vi "LINC Write Command.vi"(6 "timeout (2000)":u32=2000, 7 "parse only (F)":bool, 8 "error in (no error)":errorcluster, 9 "string command":string, 10 "packet":variant, 11 "LINC session":refnum<class "LINC.lvclass">) -> (0 "error out":errorcluster, 1 "remote error":bool, 2 "binary command":string, 3 "dup LINC session":refnum<class "LINC.lvclass">)   [LabVIEW 2018, in "STEPkgDriver_LINC.lvlib" / "LINC.lvclass"]
uses:
  LINC.lvclass
  STEPkgDriver_LINC.lvlib
  LINC Global Mode.ctl
  LINC Global Session Mode.ctl
  LINC Global Config Mode.ctl
  LINC Global Handshake Mode.ctl
  LINC Handshake Internal.ctl
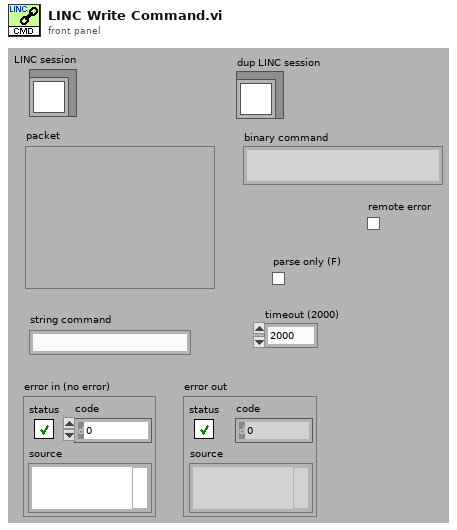
[diagram p1: front panel]
types:
  T1 = typedef "STEPkgDriver_LINC.lvlib/LINC Global Config Mode.ctl" = enum16{"INIT", "CLEAR", "SET_CMD_CB", "SET_TLM_CB", "SET_CMD_FIELDS", "SET_TLM_FIELDS", "SET_ID", "GET_CONFIG"}
  T2 = typedef "STEPkgDriver_LINC.lvlib/LINC Global Mode.ctl" = enum16{"INIT", "CLEAR", "ADD_PKT_HDR", "ADD_PKT", "GET_PKT_NAMES", "GET_PKT_DESC", "GET_PKT_HDR", "GET_PKT", "SET_PKT", "SET_DATA", "SIM_EN", "SIM_DS"}
  T3 = typedef "STEPkgDriver_LINC.lvlib/LINC Handshake Internal.ctl" = cluster{"error":errorcluster, "command data":string}
  T4 = typedef "STEPkgDriver_LINC.lvlib/LINC Global Handshake Mode.ctl" = enum16{"INIT", "CLEAR", "ADD_COMMAND", "RMV_COMMAND", "CLR_HANDSHAKE", "SET_HANDSHAKE", "GET_HANDSHAKE"}
  T5 = typedef "STEPkgDriver_LINC.lvlib/LINC Global Session Mode.ctl" = enum16{"INIT", "CLEAR", "ADD_SESSION", "SET_CONNECTION", "SET_LISTENER", "SET_REFERENCE", "GET_SESSION"}
  T6 = typedef "STEPkgDriver_LINC.lvlib/LINC Format Prototype.ctl" = cluster{"type":string, "bit offset":i32, "bit size":i32, "format":string, "unit":string, "description":string, "state values":i64[], "states":string[], "max":string, "min":string, "default":string, "array":bool, "bit element size":i32, "poly bound":dbl[], "poly scale":cluster{"coefficients":dbl[]}[], "labview size":i32, "simulate":bool, "ID":bool, "required":bool}
  T7 = typedef "STEPkgDriver_LINC.lvlib/LINC Config.ctl" = cluster{"cmd callback":refnum<vi>, "tlm callback":refnum<vi>, "cmd ID bitoffset":i32, "cmd ID bitsize":i32, "cmd IDs":i32[], "tlm ID bitoffset":i32, "tlm ID bitsize":i32, "tlm IDs":i32[], "cmd header fields":i32, "tlm header fields":i32, "tlm header size":i32}
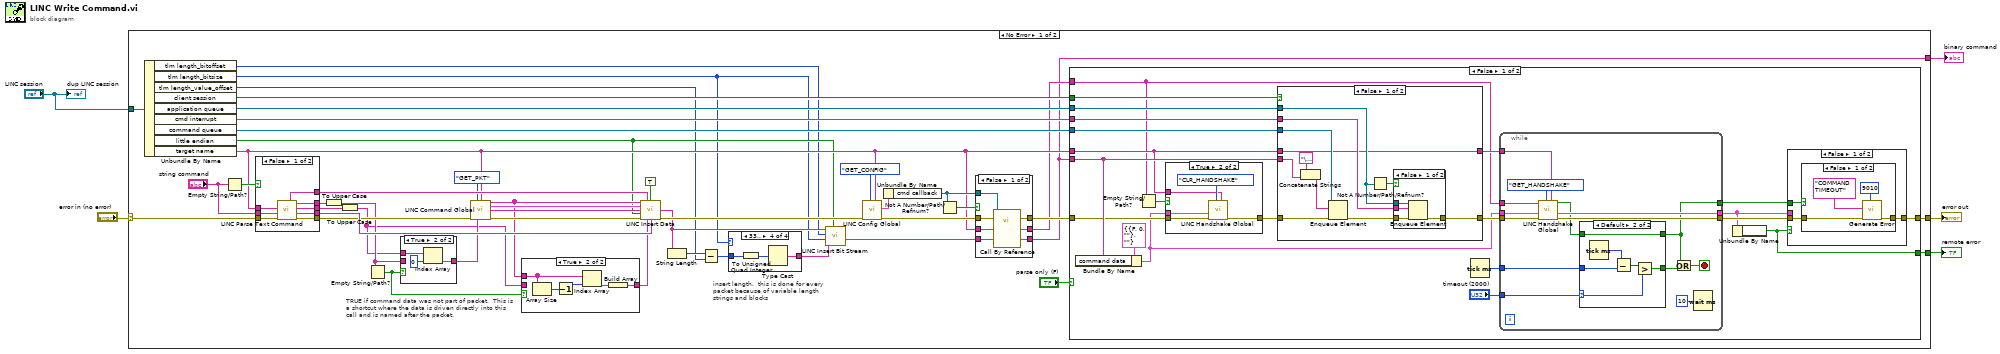
[diagram p0: block diagram]
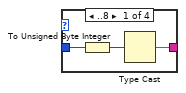
[diagram p2: hidden frame]
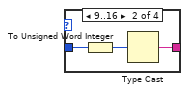
[diagram p3: hidden frame]
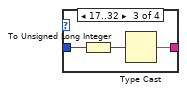
[diagram p4: hidden frame]
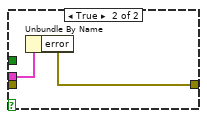
[diagram p8: hidden frame]
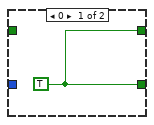
[diagram p10: hidden frame]
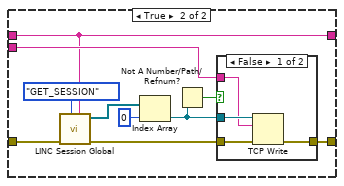
[diagram p12: hidden frame]
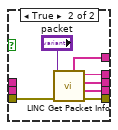
[diagram p15: hidden frame]
diagram:
  n1 = case shown="No Error" "error in (no error)" {
    selector: "error in (no error)" -> [w6 w188]
    tunnel: [w51 w188] -> w5
    tunnel: "LINC session" -> [w34 _]
    tunnel: [w19 _] -> w3
    tunnel: [w7 _] -> w2
    frame No Error {
      # "insert length.  this is done for every packet because of variable length strings and blocks"
      # "TRUE if command data was not part of packet.  This is a shortcut where the data is driven directly into this call and is named after the packet."
      n2 = Unbundle By Name(w34) -> ("tlm length_bitoffset"=w9:i32, "tlm length_bitsize"=w8:i32, "tlm length_value_offset"=w10:i32, "client session"=w33:bool, "application queue"=w32:refnum<queue>, "cmd interrupt"=w31:string, "command queue"=w30:refnum<queue>, "little endian"=w11:bool, "target name"=w22:string)
      n3 = Empty String/Path?(string/path="string command") -> (empty?=w43:bool)
      n4 = case shown="False" w43 {
        tunnel: w6 -> [w176 w183]
        tunnel: [w175 w182] -> w39
        tunnel: [w174 w180] -> w49
        tunnel: [w171 w179] -> w47
        tunnel: [w172 w178] -> w45
        tunnel: [w173 w177] -> w35
        tunnel: "string command" -> [w170 _]
        tunnel: w22 -> [w169 _]
        frame False {
          n5 = call "LINC Parse Text Command.vi"("error in (no error)"=w176, "string command"=w170, "target name"=w169) -> ("error out"=w175:errorcluster, "member data"=w174:string[], "member names"=w173:string[], "packet name"=w172:string, "member types"=w171:string[])  [unwired: 4 in]
        }
        frame True {
          n6 = call "LINC Get Packet Info.vi"("error in (no error)"=w183, "packet"="packet") -> ("error out"=w182:errorcluster, "member data"=w180:string[], "member names"=w177:string[], "packet name"=w178:string, "member types"=w179:string[])  [unwired: 5 in]
        }
      }
      n7 = To Upper Case(1:w45) -> (0:w18:string)
      n8 = To Upper Case(1:w35) -> (0:w17:string[])
      n9 = Empty String/Path?(string/path=w18) -> (empty?=w38:bool)
      n10 = case shown="True" w38 {
        tunnel: w18 -> [w184 _]
        tunnel: [w184 w185] -> w21
        tunnel: w17 -> [_ w187]
        frame False {
        }
        frame True {
          n11 = Index Array(array=w187, index=0) -> (element=w185:string)
        }
      }
      n12 = call "LINC Command Global.vi"("mode"=LINC_Global_Mode."GET_PKT", "target name"=w22, "error in (no error)"=w39, "packet name"=w21) -> ("values out"=w37:string[], "item formats out"=w48:T6[], "data out"=w40:string, "error out"=w50:errorcluster)  [unwired: 7 in, 1 out]
      n13 = case shown="True" w38 {
        tunnel: w37 -> [_ w75]
        tunnel: [w73 w74] -> w36
        tunnel: w17 -> [w73 _]
        frame False {
        }
        frame True {
          n14 = Array Size(array=w75) -> (size(s)=w76:i32)
          n15 = Decrement(x=w76) -> (x-1=w77:i32)
          n16 = Index Array(array=w75, index=w77) -> (element=w78:string)
          n17 = Build Array(w78) -> (w74:string[])
        }
      }
      n18 = call "LINC Insert Data.vi"("item names"=w37, "member types"=w47, "scale"=TRUE, "item formats"=w48, "data in"=w40, "little endian"=w11, "error in (no error)"=w50, "member names"=w36, "member data"=w49) -> ("data out"=w12:string, "error out"=w24:errorcluster)  [unwired: 5 in]
      n19 = String Length(string=w12) -> (length=w14:i32)
      n20 = Subtract(x=w14, y=w10) -> (x-y=w15:i32)
      n21 = case shown="33.." w8 {
        tunnel: w15 -> [w53 w56 w59 w62]
        tunnel: [w52 w55 w58 w61] -> w16
        frame ..8 {
          n22 = To Unsigned Byte Integer(number=w53) -> (unsigned 8bit integer=w54:u8)
          n23 = Type Cast(x=w54) -> (*(type *) &x=w52:string)  [unwired: 1 in]
        }
        frame 9..16 {
          n24 = To Unsigned Word Integer(number=w56) -> (unsigned 16bit integer=w57:u16)
          n25 = Type Cast(x=w57) -> (*(type *) &x=w55:string)  [unwired: 1 in]
        }
        frame 17..32 {
          n26 = To Unsigned Long Integer(number=w59) -> (unsigned 32bit integer=w60:u32)
          n27 = Type Cast(x=w60) -> (*(type *) &x=w58:string)  [unwired: 1 in]
        }
        frame 33.. {
          n28 = To Unsigned Quad Integer(1:w62) -> (0:w63:u64)
          n29 = Type Cast(x=w63) -> (*(type *) &x=w61:string)  [unwired: 1 in]
        }
      }
      n30 = call "LINC Insert Bit Stream.vi"("little endian"=w11, "data to insert"=w16, "bit size"=w8, "bit offset"=w9, "data in"=w12) -> ("data out"=w13:string)  [unwired: 4 in]
      n31 = call "LINC Config Global.vi"("target name"=w22, "mode"=LINC_Global_Config_Mode."GET_CONFIG", "error in (no error)"=w24) -> ("error out"=w26:errorcluster, "config out"=w25:T7)  [unwired: 7 in]
      n32 = Unbundle By Name(w25) -> ("cmd callback"=w28:refnum<vi>)
      n33 = Not A Number/Path/Refnum?(number/path/refnum=w28) -> (NaN/Path/Refnum?=w27:bool)
      n34 = case shown="False" w27 {
        tunnel: [w70 w72] -> w23
        tunnel: w13 -> [w69 w71]
        tunnel: [w68 w71] -> w19
        tunnel: w26 -> [w67 w72]
        tunnel: w28 -> [w66 _]
        tunnel: w22 -> [w65 _]
        tunnel: [w64 _] -> w20
        frame False {
          n35 = call-by-ref "?"(reference=w66, error in=w67, "command in"=w69, "target name"=w65) -> (error out=w70:errorcluster, "command out"=w68:string, "GUID"=w64:string)  [unwired: 1 out]
        }
        frame True {
        }
      }
      n36 = case shown="False" "parse only (F)" {
        tunnel: [w81 w168] -> w51
        tunnel: w30 -> [w99 _]
        tunnel: w23 -> [w89 w168]
        tunnel: w19 -> [w90 _]
        tunnel: w31 -> [w98 _]
        tunnel: w32 -> [w97 _]
        tunnel: w33 -> [w96 _]
        tunnel: w22 -> [w87 _]
        tunnel: w20 -> [w85 _]
        tunnel: [w79 _] -> w7
        frame False {
          n37 = Bundle By Name(cluster=T3 {"error"={"status"=FALSE, "code"=0, "source"=""}, "command data"=""} ("handshake in"), "command data"=w90) -> (w86:T3)
          n38 = Empty String/Path?(string/path=w85) -> (empty?=w84:bool)
          n39 = case shown="True" w84 {
            tunnel: w89 -> [w110 w114]
            tunnel: [w110 w113] -> w88
            tunnel: w87 -> [_ w112]
            tunnel: w86 -> [_ w111]
            frame False {
            }
            frame True {
              n40 = call "LINC Handshake Global.vi"("target name"=w112, "mode"=LINC_Global_Handshake_Mode."CLR_HANDSHAKE", "error in (no error)"=w114, "handshake in"=w111) -> ("error out"=w113:errorcluster)  [unwired: 4 in, 3 out]
            }
          }
          n41 = case shown="False" w96 {
            tunnel: w99 -> [w147 _]
            tunnel: w88 -> [w145 w153]
            tunnel: w90 -> [w144 w159]
            tunnel: [w140 w162] -> w95
            tunnel: w98 -> [w139 _]
            tunnel: w97 -> [w138 _]
            tunnel: w87 -> [w137 w154]
            tunnel: [w137 w154] -> w94
            frame False {
              n42 = Concatenate Strings("\u0001" ("string"), w144) -> (w146:string)
              n43 = Enqueue Element(queue=w147, element=w146, error in (no error)=w145) -> (error out=w141:errorcluster)  [unwired: 1 in, 2 out]
              n44 = Not A Number/Path/Refnum?(number/path/refnum=w138) -> (NaN/Path/Refnum?=w142:bool)
              n45 = case shown="False" w142 {
                tunnel: w141 -> [w151 w152]
                tunnel: [w150 w152] -> w140
                tunnel: w138 -> [w149 _]
                tunnel: w139 -> [w148 _]
                frame False {
                  n46 = Enqueue Element(queue=w149, element=w148, error in (no error)=w151) -> (error out=w150:errorcluster)  [unwired: 1 in, 2 out]
                }
                frame True {
                }
              }
            }
            frame True {
              n47 = call "LINC Session Global.vi"("target name"=w154, "mode"=LINC_Global_Session_Mode."GET_SESSION", "error in (no error)"=w153) -> ("error out"=w161:errorcluster, "connections out"=w157:refnum<k5>[])  [unwired: 4 in, 3 out]
              n48 = Index Array(array=w157, index=0) -> (element=w155:refnum<k5>)
              n49 = Not A Number/Path/Refnum?(number/path/refnum=w155) -> (NaN/Path/Refnum?=w160:bool)
              n50 = case shown="False" w160 {
                tunnel: [w166 w167] -> w162
                tunnel: w161 -> [w165 w167]
                tunnel: w155 -> [w164 _]
                tunnel: w159 -> [w163 _]
                frame False {
                  n51 = TCP Write(connection ID=w164, data in=w163, error in (no error)=w165) -> (error out=w166:errorcluster)  [unwired: 1 in, 2 out]
                }
                frame True {
                }
              }
            }
          }
          n52 = Tick Count (ms)() -> (millisecond timer value=w93:u32)
          n53 = while {
            tunnel: w95 -> [w128]
            tunnel: [w127] -> w83
            tunnel: w94 -> [w126]
            tunnel: w85 -> [w125]
            tunnel: w93 -> [w124]
            tunnel: "timeout (2000)" -> [w121]
            tunnel: [w116] -> w80
            tunnel: w86 -> [w119]
            tunnel: [w118] -> w82
            stop <- w122 stop-if-true
            n54 = call "LINC Handshake Global.vi"("target name"=w126, "mode"=LINC_Global_Handshake_Mode."GET_HANDSHAKE", "error in (no error)"=w128, "handshake in"=w119, "GUID"=w125) -> ("error out"=w127:errorcluster, "handshake out"=w118:T3, "handshake"=w117:bool)  [unwired: 3 in, 1 out]
            n55 = case shown="Default" w121 {
              selector: w121 -> [_ w132]
              tunnel: w124 -> [_ w136]
              tunnel: [w130 w133] -> w120
              tunnel: w117 -> [_ w131]
              tunnel: [w130 w131] -> w116
              frame 0 {
                w130 = TRUE
              }
              frame Default {
                n56 = Tick Count (ms)() -> (millisecond timer value=w135:u32)
                n57 = Subtract(x=w135, y=w136) -> (x-y=w134:u32)
                n58 = Greater?(x=w134, y=w132) -> (0:w133:bool)
              }
            }
            n59 = Or(x=w116, y=w120) -> (x .or. y?=w122:bool)
            n60 = Wait (ms)(milliseconds to wait=u32 10) -> ()  [unwired: 1 out]
          }
          n61 = Unbundle By Name(w82) -> ("error.status"=w79:bool)
          n62 = case shown="False" w79 {
            tunnel: w83 -> [w102 _]
            tunnel: w82 -> [_ w109]
            tunnel: [w100 w108] -> w81
            tunnel: w80 -> [w101 _]
            frame False {
              n63 = case shown="False" w101 {
                tunnel: w102 -> [w106 w107]
                tunnel: [w105 w107] -> w100
                frame False {
                  n64 = call "Generate Error.vi"("error code (-1301)"=9010, "error in"=w106, "description"="COMMAND TIMEOUT") -> ("error out"=w105:errorcluster)  [unwired: 8 in]
                }
                frame True {
                }
              }
            }
            frame True {
              n65 = Unbundle By Name(w109) -> ("error"=w108:errorcluster)
            }
          }
        }
        frame True {
        }
      }
    }
    frame Error {
    }
  }
  "error out" <- w5
  "binary command" <- w3
  "remote error" <- w2
  "dup LINC session" <- "LINC session"
